vi "AB_Engine_Compute_PackedLib_Implied_Links.vi"(9 "links in":u32[](array[numeric]), 11 "Linker:Read Info From File":T2(array[cluster])) -> (1 "links out":u32[](array[numeric]))   [LabVIEW 2020]
doc: "This VI adds all owned instance VI and private data control links to our links (recursively), and checks to see if ourselves or any VI whose links we are assuming require us to keep our front panel"
uses:
  <vilib>/Utility/lvfile.llb/LVFileType.ctl
  <vilib>/Utility/lvfile.llb/NI_FileType.lvlib
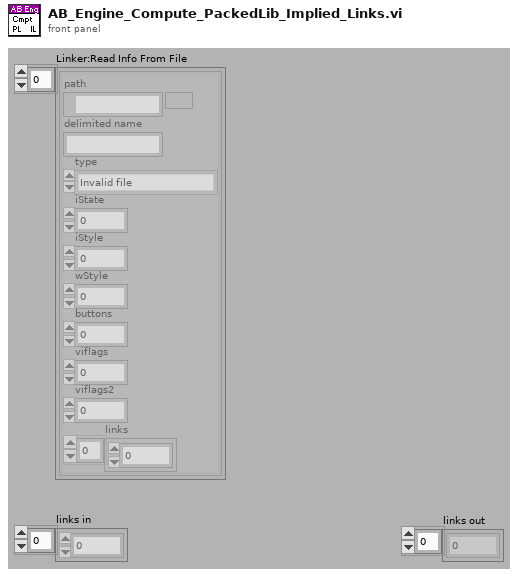
[diagram p1: front panel]
types:
  T1 = typedef "NI_FileType.lvlib/LVFileType.ctl" = enum32{"Invalid file", "Unknown type", "Instrument", "Control", "Polymorphic VI", "Project", "Library", "LVClass", "XControl", "XNode", "Shared library", ".NET assembly", "ActiveX interface", "CIN", "Run-time menu", "Palette menu", "Help file", "LLB", "XNode Edit Dependency", "Class Private Data Control", "Statechart", "MathScript .m file", "Ladder Diagram", "LVLibp", "XNode Build Dependency"}
  T2 = cluster{"path":path, "delimited name":string, "type":T1, "iState":u32, "iStyle":u16, "wStyle":u16, "buttons":u16, "viflags":u32, "viflags2":u32, "links":u32[]}[]
  T3 = cluster{"path":path, "delimited name":string, "type":T1, "iState":u32, "iStyle":u16, "wStyle":u16, "buttons":u16, "viflags":u32, "viflags2":u32, "links":u32[]}
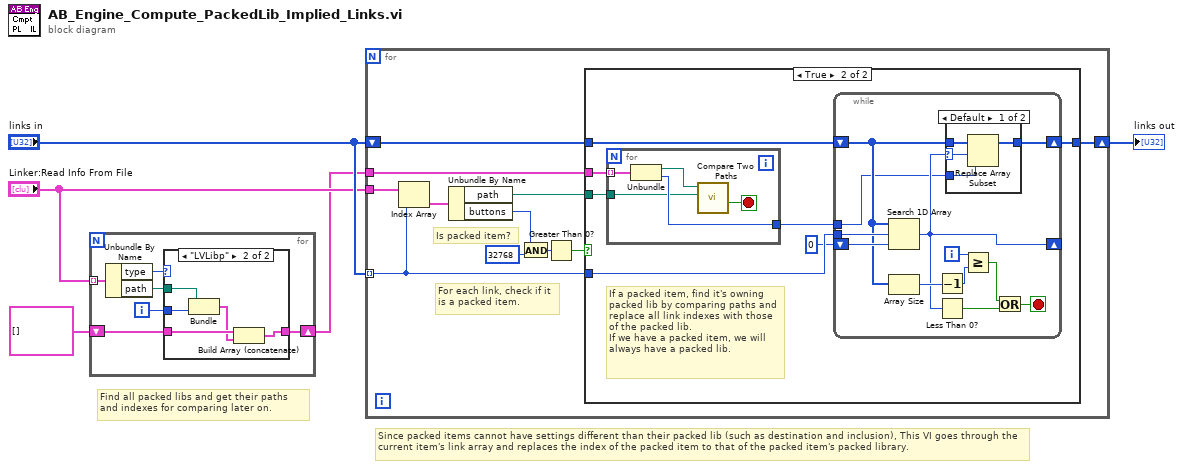
[diagram p0: block diagram]
diagram:
  # "Find all packed libs and get their paths and indexes for comparing later on."
  # "Since packed items cannot have settings different than their packed lib (such as destination and inclusion), This VI goes through the current item's link array and replaces the index of the packed item to that of the packed item's packed library."
  n1 = for {
    tunnel: "Linker:Read Info From File" -> [w11] mode=indexing
    shift-right: [w6] -> w1
    shift-left: cluster{"path":path, i32}[] [] -> [w7]
    i -> [w8]
    n2 = Unbundle By Name(w11) -> ("type"=w10:T1, "path"=w9:path)
    n3 = case shown="\"LVLibp\"" w10 {
      tunnel: w9 -> [_ w17]
      tunnel: w8 -> [_ w16]
      tunnel: w7 -> [w12 w15]
      tunnel: [w12 w13] -> w6
      frame Default {
      }
      frame "LVLibp" {
        n4 = Bundle("path"=w17, w16) -> (w14:cluster{"path":path, i32})  [unwired: 1 in]
        n5 = Build Array (concatenate)(w15, w14) -> (w13:cluster{"path":path, i32}[])
      }
    }
  }
  n6 = for {
    tunnel: "links in" -> [w27] mode=indexing
    tunnel: "Linker:Read Info From File" -> [w21]
    shift-right: [w20] -> w5
    shift-left: "links in" -> [w28]
    tunnel: w1 -> [w19]
    # "For each link, check if it is a packed item."
    # "Is packed item?"
    n7 = Index Array(array=w21, index=w27) -> (element=w23:T3)
    n8 = Unbundle By Name(w23) -> ("path"=w18:path, "buttons"=w26:u16)
    n9 = And(x=w26, y=u16 32768) -> (x .and. y?=w24:u16)
    n10 = Greater Than 0?(x=w24) -> (x > 0?=w22:bool)
    n11 = case shown="True" w22 {
      tunnel: w28 -> [w29 w36]
      tunnel: w27 -> [_ w35]
      tunnel: w19 -> [_ w30]
      tunnel: [w29 w32] -> w20
      tunnel: w18 -> [_ w31]
      frame False {
      }
      frame True {
        # "If a packed item, find it's owning packed lib by comparing paths and replace all link indexes with those of the packed lib.\nIf we have a packed item, we will always have a packed lib."
        n12 = for {
          tunnel: [w57] -> w34
          tunnel: w31 -> [w54]
          tunnel: w30 -> [w58] mode=indexing
          stop <- w56 stop-if-true
          n13 = Unbundle(w58) -> ("path"=w55:path, w57:i32)
          n14 = call <vilib>:"Compare Two Paths.vi"("Path 2"=w54, "Path 1"=w55) -> ("Path 2 Relative to Path 1?"=w56:bool)  [unwired: 6 in, 3 out]
        }
        n15 = while {
          shift-right: [w38] -> w32
          shift-left: w36 -> [w39]
          tunnel: w35 -> [w48]
          tunnel: w34 -> [w37]
          shift-right: [w40] -> _
          shift-left: 0 ("index of element") -> [w41]
          i -> [w44]
          stop <- w46 stop-if-true
          n16 = Search 1D Array(1D array=w39, element=w48, start index (0)=w41) -> (index of element=w40:i32)
          n17 = Array Size(array=w39) -> (size(s)=w45:i32)
          n18 = Decrement(x=w45) -> (x-1=w43:i32)
          n19 = Less Than 0?(x=w40) -> (x < 0?=w47:bool)
          n20 = case shown="Default" w40 {
            selector: w40 -> [w50 _]
            tunnel: [w51 w53] -> w38
            tunnel: w39 -> [w52 w53]
            tunnel: w37 -> [w49 _]
            frame Default {
              n21 = Replace Array Subset(array=w52, new element=w49, index=w50) -> (w51:u32[])
            }
            frame -1 {
            }
          }
          n22 = Greater Or Equal?(x=w44, y=w43) -> (x >= y?=w42:bool)
          n23 = Or(x=w42, y=w47) -> (x .or. y?=w46:bool)
        }
      }
    }
  }
  "links out" <- w5
